vi "WSVCAP SHL Host LL I2C Convert Channel Bytes to Bit Array.vi"(0 "C1 Data Out":u8[][](array[numeric]) format="%.0x") -> (4 "Write Data":u64[](array[numeric]) format="%032b")   [LabVIEW 2017]
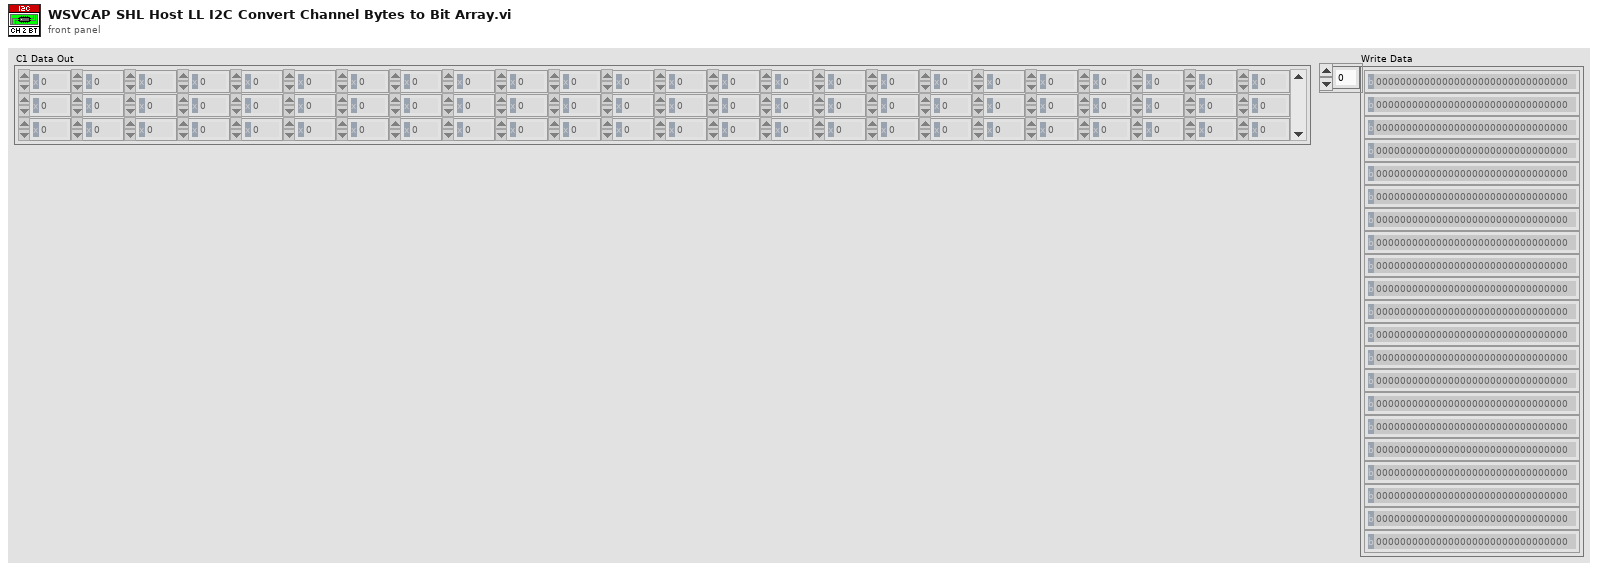
[diagram p1: front panel]
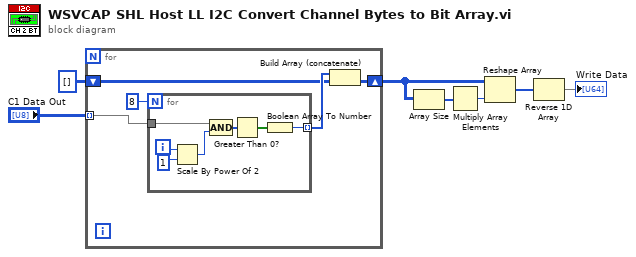
[diagram p0: block diagram]
diagram:
  n1 = for {
    tunnel: "C1 Data Out" -> [w8] mode=indexing
    shift-right: [w10] -> w1
    shift-left: u64[][] [] -> [w9]
    n2 = for {
      N: 8 -> [_]
      tunnel: w8 -> [w15]
      tunnel: [w14] -> w11 mode=indexing
      i -> [w17]
      n3 = Scale By Power Of 2(n=w17, x=u8 1) -> (x*2^n=w18:u8)
      n4 = Compound Arithmetic op=AND(w15, w18) -> (w19:u8[])
      n5 = Greater Than 0?(x=w19) -> (x > 0?=w13:bool[])
      n6 = Boolean Array To Number(Boolean array=w13) -> (number=w14:u64)
    }
    n7 = Build Array (concatenate)(w11, w9) -> (w10:u64[][])
  }
  n8 = Array Size(array=w1) -> (size(s)=w6:i32[])
  n9 = Multiply Array Elements(1:w6) -> (0:w5:i32)
  n10 = Reshape Array(w1, w5) -> (w4:u64[])
  n11 = Reverse 1D Array(array=w4) -> (reversed array=→"Write Data":u64[])
